vi "Neutral_Agilent_CheckForChange_20170616.vi"(0 "Control Reference Cluster Input":T8, 1 "Scan Parameters":T1={"Initial Values"=[81.5, 1.0, -0.1, 1.0], "Final Values"=[82.5, 3.0, 0.075, 5.0], "Step Sizes"=[0.015, 1.0, 0.025, 1.0], "Parameters to Change"=[enum."Synth Frequency", enum."Dummy Variable", enum."Red Mot 87 Initial Voltage", enum."Dummy Variable"], "Channels to Change"=[2, 0, 7, 0], "Number of Parameters to Scan"=2, "Parameter Nickname (no spaces)"=["", "ScanNo-", "Z-", "ScanNo-"], "Scan Base Name"="88Sr_3P1Spec_BFieldZero_X-0.02A_Y-0.277A_Z-0.6A_", "Raw_Data Folder"=path "\\\\mercury\\Neutral_Experiment/Raw_Data/2017.06.15", "ROI Parameters"={"Background Radius"=150.0, "Atom Radius"=120.0, "X Center"=365.0, "Y Center"=460.0}, "Drop Time (ms)"=17.0, "Phases To Change"=[1, 0, 2, 0], "Scan Pulseblaster Channel With Parameter"={"Change PB Time Toggle"=FALSE, "PB Channel"=10.0, "Parameter Number"=0.0}, "Preserve Waveform\nContinuity"=FALSE, "Generated Array Type"=enum."Default (old way)", "Master Batch Third Column"=0.277, "Master Batch Fourth Column"=0.0, "Master Batch Fifth Column"=0.0, "Current Param. Values"=[81.5, 1.0]} {"Current Param. Values" format="%^#.3e"; "Drop Time (ms)" min=1.0; "Number of Parameters to Scan" min=1}, 2 "Auto Program Agilent":bool, 3 "error in (no error)":errorcluster) -> (7 "Changed Current?":bool, 10 "Error Out":errorcluster)   [LabVIEW 2016]
uses:
  Controls/Agilent E3631A/Settings_Control.ctl
  Controls/Agilent E3631A/Measurement_Indicator.ctl
  Controls/Agilent E3631A/Trigger_Settings.ctl
  Controls/ScanParameters/ScanParametersPanel.ctl
  Controls/ScanParameters/ParameterToChange.ctl
  Controls/ScanParameters/ROI_set.ctl
  Controls/ScanParameters/ScanPBandParam.ctl
panel:
  in  "Agilent E3631A Settings":T5={"VISA resource name"="GPIB0::5::INSTR", "Voltage Set (6V max)"=6.0, "Current Set (5A max)"=0.007, "Voltage Set (25V max)"=25.0, "Current Set (1A max)"=0.225, "Voltage Set (-25V max)"=25.0, "Current Set (1A max)"=0.225, "6V Switch"=FALSE, "+25V Switch"=FALSE, "-25V Switch"=FALSE, "Agilent E3631A Measurements"={"6V Actual Voltage Level (V)"=0.03231557, "6V Actual Current Level (A)"=0.01701259, "25V Actual Voltage Level (V)"=0.4256878, "25V Actual Current Level (A)"=0.2772881, "-25V Actual Current Level (A)"=0.0, "-25V Actual Voltage Level (V)"=0.0}, "Triggered Agilent Settings"={"Trigger \nDelay (s)"=3.0, "Enable +6V Channel"=TRUE, "+6V Current"=0.02, "Enable -25V Channel"=FALSE, "-25V Current"=0.0, "Enable +25V Channel"=TRUE, "+25V Current"=0.275}, "Auto Program Agilent"=FALSE, "Agilent Software Trigger"=FALSE} {"Triggered Agilent Settings"."Trigger \nDelay (s)" min=0.0 max=3600.0 step=1.0 format="%.2f"; "Agilent E3631A Measurements"."-25V Actual Current Level (A)" format="%.3g"; "Agilent E3631A Measurements"."-25V Actual Voltage Level (V)" format="%.3g"; "Agilent E3631A Measurements"."25V Actual Current Level (A)" format="%.3g"; "Agilent E3631A Measurements"."25V Actual Voltage Level (V)" format="%.3g"; "Agilent E3631A Measurements"."6V Actual Current Level (A)" format="%.3g"; "Agilent E3631A Measurements"."6V Actual Voltage Level (V)" format="%.3g"; "Current Set (1A max)" format="%.3g"; "Voltage Set (-25V max)" format="%.3g"; "Current Set (1A max)" format="%.3g"; "Voltage Set (25V max)" format="%.3g"; "Current Set (5A max)" format="%.3g"; "Voltage Set (6V max)" format="%.3g"}
  # "Select a PB Channel to set with a phase time for evaporation or whatever"
  # "Since the Agilent is slow to communicate the program will skip programming if the \"Auto Program Agilent\" switch is disabled.  If \"Auto Program\" is enabled the settings to the far left are used to program the Agilent.\n\nAdditionally, the Agilent has an internal software trigger that can a single channel between two current setpoints. The clock is not referenced to the Pulseblaster so be careful with timing when using the Triggered Agilent Settings. To enabled this mode use the \"Agilent Software Trigger\" swithc.\n\nUse the \"Program Agilent\" button to perform a one-time write (with settings on the far left) to avoid having the slow response of the supply during data scans.\n\nNOTE: When setting only current values the program will default to setting the maximum allowed voltage for a given channel."
  # "6V (2017.06.15)\n\nReported Current = \nSet Cur - 0.003A\n\nActual Current = \nSet Cur - 0.0015A"
  # "+25V (2017.06.15)\n\nReported Current = \nSet Cur + 0.002A\n\nActual Current = \nSet Cur + 0.002A"
  # "-25V (2017.06.15)\n\nReported Current = \nSet Cur\n\nActual Current = \nSet Cur"
  # "Beware of the offset in set, reported and actual current from Agilent channels. Below are corrections measured for each channel"
  # "--25V  Measurements"
  # "+25V  Measurements"
  # "6V  Measurements"
  # "-25V Output Settings"
  # "+25V Output Settings"
  # "6V Output Settings"
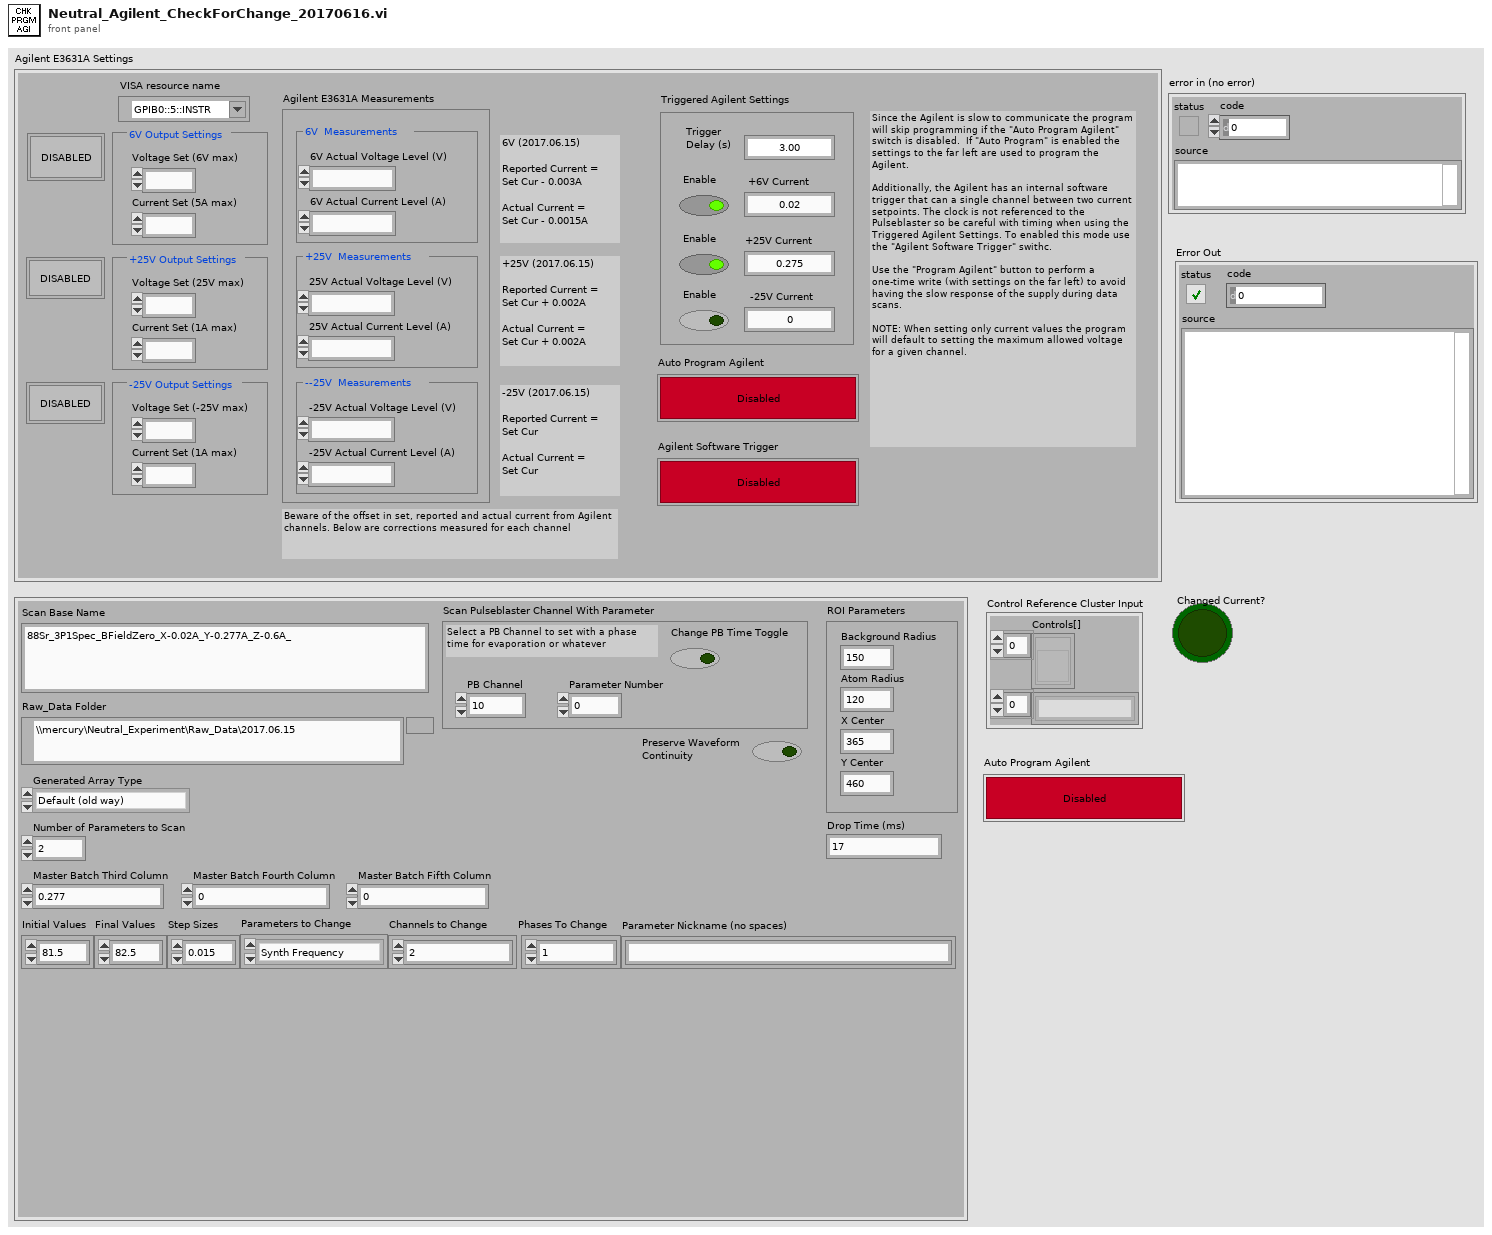
[diagram p1: front panel]
types:
  T1 = typedef "ScanParametersPanel.ctl" = cluster{"Initial Values":dbl[], "Final Values":dbl[], "Step Sizes":dbl[], "Parameters to Change":T2[], "Channels to Change":u32[], "Number of Parameters to Scan":i32, "Parameter Nickname (no spaces)":string[], "Scan Base Name":string, "Raw_Data Folder":path, "ROI Parameters":T3, "Drop Time (ms)":dbl, "Phases To Change":u32[], "Scan Pulseblaster Channel With Parameter":T4, "Preserve Waveform\nContinuity":bool, "Generated Array Type":enum16{"Custom Array From File", "Default (old way)"}, "Master Batch Third Column":dbl, "Master Batch Fourth Column":dbl, "Master Batch Fifth Column":dbl, "Current Param. Values":dbl[]}
  T2 = typedef "ParameterToChange.ctl" = enum16{"Dummy Variable", "Synth Amplitude", "Synth Frequency", "Synth Phase", "ODT Params Phase Time", "ODT Params Tau", "ODT Params Final Voltage", "ODT Params Initial Voltage", "ODT Params Eta", "Red Mot 88 Phase Time", "Red Mot 87 Phase Time", "Red Mot 88 Final Voltage", "Red Mot 88 Initial Voltage", "Red Mot 87 Final Voltage", "Red Mot 87 Initial Voltage", "PulseBlaster", "6713 Voltage", "Green Lattice Phase Time", "Green Lattice Initial Voltage", "Green Lattice Final Voltage", "Agilent Current Setpoint", "FPGA - Constant Op - Set", "FPGA - Bool Op - Output HI", "FPGA - Bool Op - Output LO", "FPGA - Custom Op"}
  T3 = typedef "ROI_set.ctl" = cluster{"Background Radius":dbl, "Atom Radius":dbl, "X Center":dbl, "Y Center":dbl}
  T4 = typedef "ScanPBandParam.ctl" = cluster{"Change PB Time Toggle":bool, "PB Channel":dbl, "Parameter Number":dbl}
  T5 = typedef "Settings_Control.ctl" = cluster{"VISA resource name":refnum<visa-resource-name>, "Voltage Set (6V max)":dbl, "Current Set (5A max)":dbl, "Voltage Set (25V max)":dbl, "Current Set (1A max)":dbl, "Voltage Set (-25V max)":dbl, "Current Set (1A max)":dbl, "6V Switch":bool, "+25V Switch":bool, "-25V Switch":bool, "Agilent E3631A Measurements":T6, "Triggered Agilent Settings":T7, "Auto Program Agilent":bool, "Agilent Software Trigger":bool}
  T6 = typedef "Measurement_Indicator.ctl" = cluster{"6V Actual Voltage Level (V)":dbl, "6V Actual Current Level (A)":dbl, "25V Actual Voltage Level (V)":dbl, "25V Actual Current Level (A)":dbl, "-25V Actual Current Level (A)":dbl, "-25V Actual Voltage Level (V)":dbl}
  T7 = typedef "Trigger_Settings.ctl" = cluster{"Trigger \nDelay (s)":dbl, "Enable +6V Channel":bool, "+6V Current":dbl, "Enable -25V Channel":bool, "-25V Current":dbl, "Enable +25V Channel":bool, "+25V Current":dbl}
  T8 = cluster{"Controls[]":refnum<vi>[], "Control Names":string[]}
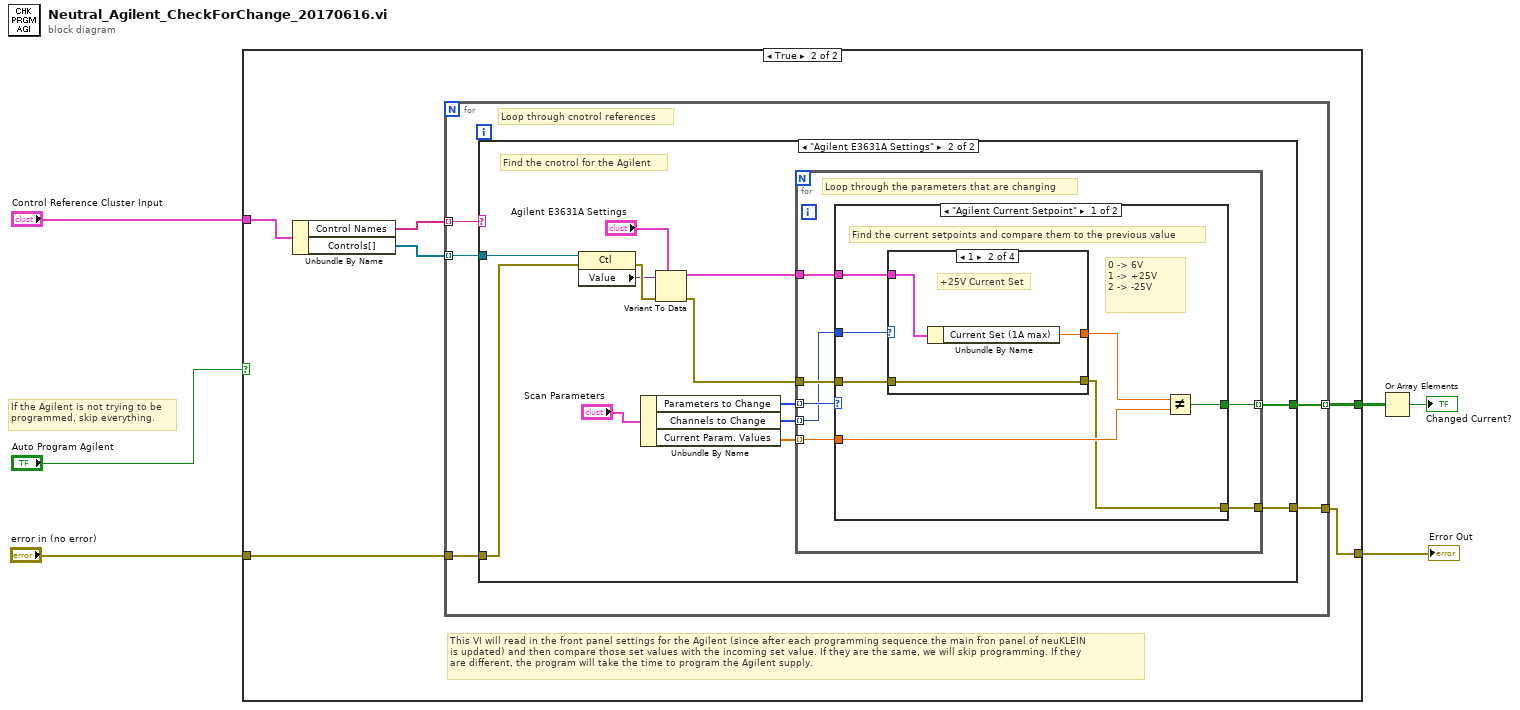
[diagram p0: block diagram]
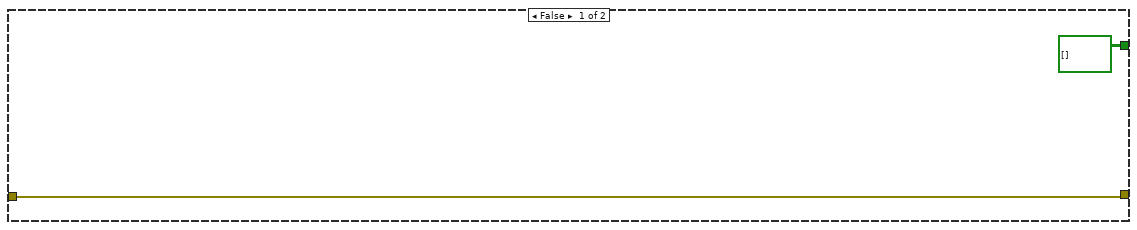
[diagram p2: hidden frame]
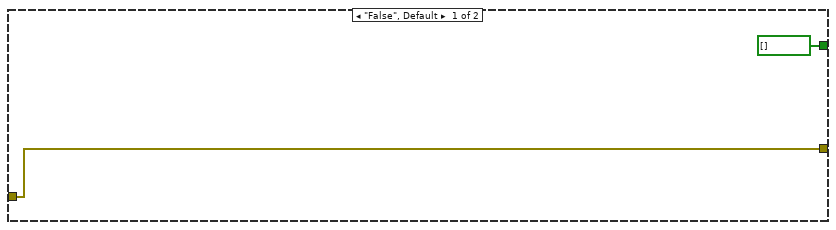
[diagram p3: hidden frame]
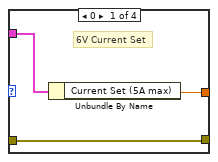
[diagram p4: hidden frame]
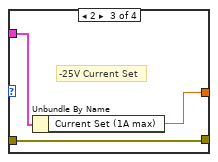
[diagram p5: hidden frame]
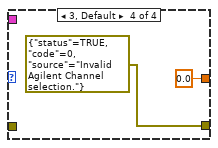
[diagram p6: hidden frame]
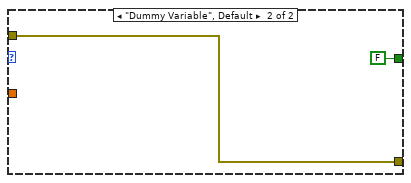
[diagram p7: hidden frame]
diagram:
  # "If the Agilent is not trying to be\nprogrammed, skip everything."
  n1 = case shown="True" "Auto Program Agilent" {
    tunnel: "error in (no error)" -> [w7 w12]
    tunnel: [w7 w11] -> w5
    tunnel: "Control Reference Cluster Input" -> [_ w10]
    tunnel: [bool[][] [] w9] -> w2
    frame False {
    }
    frame True {
      # "This VI will read in the front panel settings for the Agilent (since after each programming sequence the main fron panel of neuKLEIN\nis updated) and then compare those set values with the incoming set value. If they are the same, we will skip programming. If they\nare different, the program will take the time to program the Agilent supply."
      n2 = Unbundle By Name(w10) -> ("Control Names"=w13:string[], "Controls[]"=w14:refnum<vi>[])
      n3 = for {
        tunnel: w13 -> [w19] mode=indexing
        tunnel: w14 -> [w18] mode=indexing
        tunnel: w12 -> [w17]
        tunnel: [w16] -> w11
        tunnel: [w15] -> w9 mode=indexing
        # "Loop through cnotrol references"
        n4 = case shown="\"Agilent E3631A Settings\"" w19 {
          tunnel: w18 -> [_ w31]
          tunnel: w17 -> [w21 w30]
          tunnel: [w21 w24] -> w16
          tunnel: [bool[] [] w23] -> w15
          frame "False", Default {
          }
          frame "Agilent E3631A Settings" {
            # "Find the cnotrol for the Agilent"
            n5 = property class="Ctl"(reference=w31, error in=w30) -> (error out=w34:errorcluster, "Value"=w33:variant)  [unwired: 1 out]
            n6 = Unbundle By Name("Scan Parameters") -> ("Parameters to Change"=w28:T2[], "Channels to Change"=w22:u32[], "Current Param. Values"=w26:dbl[])
            n7 = Variant To Data(error in=w34, type="Agilent E3631A Settings", Variant=w33) -> (data=w27:T5, error out=w25:errorcluster)
            n8 = for {
              tunnel: w28 -> [w41] mode=indexing
              tunnel: w27 -> [w40]
              tunnel: w26 -> [w39] mode=indexing
              tunnel: w25 -> [w38]
              tunnel: [w37] -> w24
              tunnel: [w36] -> w23 mode=indexing
              tunnel: w22 -> [w35] mode=indexing
              # "Loop through the parameters that are changing"
              n9 = case shown="\"Agilent Current Setpoint\"" w41 {
                tunnel: w40 -> [w48 _]
                tunnel: w39 -> [w46 _]
                tunnel: w38 -> [w45 w60]
                tunnel: [w44 w60] -> w37
                tunnel: [w43 FALSE] -> w36
                tunnel: w35 -> [w42 _]
                frame "Agilent Current Setpoint" {
                  # "Find the current setpoints and compare them to the previous value"
                  # "0 -> 6V\n1 -> +25V\n2 -> -25V"
                  n10 = case shown="1" w42 {
                    tunnel: [w51 w54 w57 errorcluster {"status"=TRUE, "code"=0, "source"="Invalid Agilent Channel selection."} ("error constant")] -> w44
                    tunnel: w45 -> [w51 w54 w57 _]
                    tunnel: w48 -> [w50 w53 w56 _]
                    tunnel: [w49 w52 w55 0.0 ("Current Set (1A max)")] -> w47
                    frame 0 {
                      # "6V Current Set"
                      n11 = Unbundle By Name(w50) -> ("Current Set (5A max)"=w49:dbl)
                    }
                    frame 1 {
                      # "+25V Current Set"
                      n12 = Unbundle By Name(w53) -> ("Current Set (1A max)"=w52:dbl)
                    }
                    frame 2 {
                      # "-25V Current Set"
                      n13 = Unbundle By Name(w56) -> ("Current Set (1A max)"=w55:dbl)
                    }
                    frame 3, Default {
                    }
                  }
                  n14 = Not Equal?(x=w47, y=w46) -> (x != y?=w43:bool)
                }
                frame "Dummy Variable", Default {
                }
              }
            }
          }
        }
      }
    }
  }
  "Error Out" <- w5
  n15 = Or Array Elements(Boolean array=w2) -> (logical OR=→"Changed Current?":bool)
